vi "proceed.vi"(8 "error in (no error)":errorcluster, 11 "ScanModeDL091001Scaffold in":refnum<class "ImagingModeDL100901FlexTrajectory.lvclass">) -> (0 "error out":errorcluster, 3 "ScanModeDL091001Scaffold out":refnum<class "ImagingModeDL100901FlexTrajectory.lvclass">)   [LabVIEW 2010, in "ImagingModeDL100901FlexTrajectory.lvclass"]
uses:
  ImagingModeDL100901FlexTrajectory.lvclass
  ImagingModeDL100901FlexTrajectory.lvclass/ImagingModeDL100901FlexTrajectory.ctl
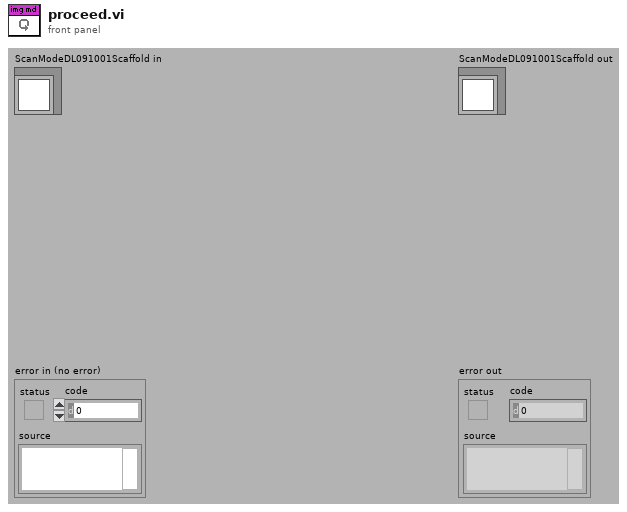
[diagram p1: front panel]
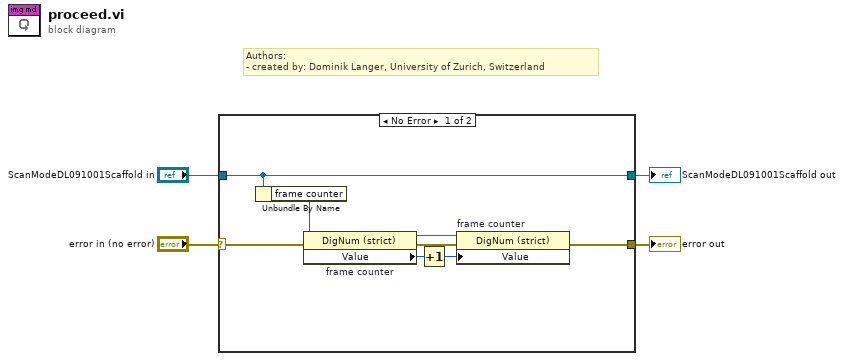
[diagram p0: block diagram]
diagram:
  # "Authors: \n- created by: Dominik Langer, University of Zurich, Switzerland"
  n1 = case shown="No Error" "error in (no error)" {
    selector: "error in (no error)" -> [w6 w14]
    tunnel: [w8 w14] -> w3
    tunnel: [w5 w13] -> w2
    tunnel: "ScanModeDL091001Scaffold in" -> [w5 w13]
    frame No Error {
      n2 = Unbundle By Name(w5) -> ("frame counter"=w12:refnum<vi>)
      n3 = property on="frame counter" class="DigNum (strict)"(reference=w12, error in=w6) -> (reference out=w10:refnum<vi>, error out=w9:errorcluster, "Value"=w11:i32)
      n4 = Increment(x=w11) -> (x+1=w7:i32)
      n5 = property on="frame counter" class="DigNum (strict)"(reference=w10, error in=w9, "Value"=w7) -> (error out=w8:errorcluster)  [unwired: 1 out]
    }
    frame Error {
    }
  }
  "error out" <- w3
  "ScanModeDL091001Scaffold out" <- w2
